vi "PolhemusTesting.vi"() -> ()   [LabVIEW 2009]
panel:
  out "roll":sgl format="%8.1f"
  out "el":sgl format="%8.1f"
  out "az":sgl format="%8.1f"
  in  "stop":bool
  out "z":sgl format="%8.1f"
  out "y":sgl format="%8.1f"
  out "x":sgl format="%8.1f"
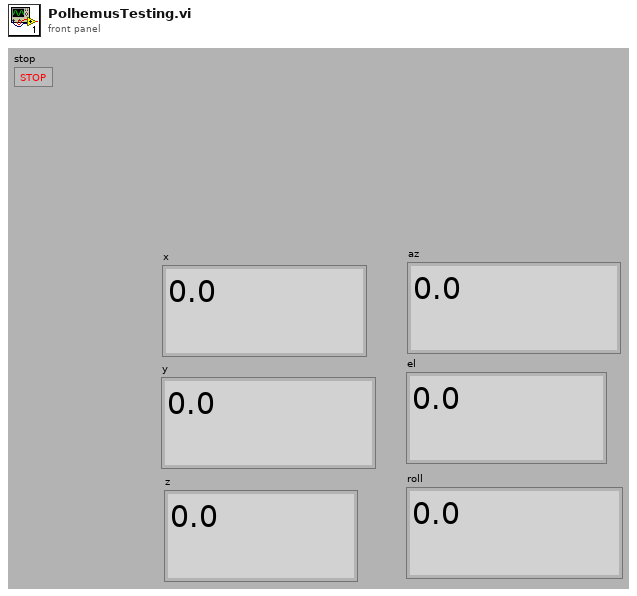
[diagram p1: front panel]
types:
  T1 = cluster{"#Bytes":i32[], "Titles":string[], "Format":enum16{"ASCII", "Binary"}, "Units":enum16{"Inches", "Centimeters"}, "Station State":bool[], "#Line Feeds":i32}
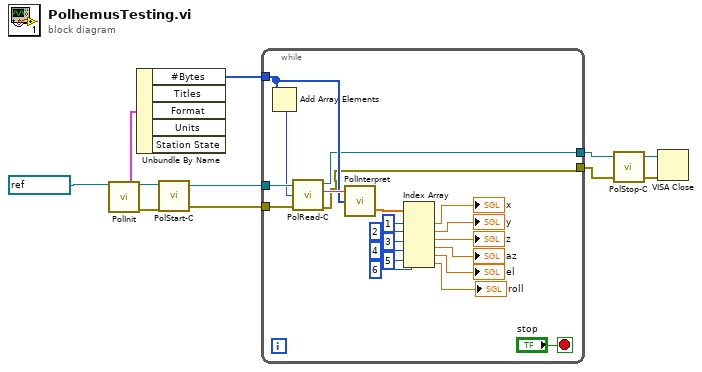
[diagram p0: block diagram]
diagram:
  n1 = call "PolInit.vi"("VISA resource name"=refnum<visa-resource-name> "COM3") -> ("VISA resource name out"=w9:refnum<visa-resource-name>, "Polhemus Info"=w10:T1, "error out"=w8:errorcluster)  [unwired: 12 in]
  n2 = Unbundle By Name(w10) -> ("#Bytes"=w5:i32[])  [unwired: 4 out]
  n3 = call "PolStart-C.vi"("error in (no error)"=w8, "VISA resource name"=w9) -> ("error out"=w6:errorcluster, "VISA resource name out"=w7:refnum<visa-resource-name>)  [unwired: 2 in]
  n4 = while {
    tunnel: w7 -> [w32]
    tunnel: w6 -> [w31]
    tunnel: w5 -> [w28]
    tunnel: [w20] -> w4
    tunnel: [w19] -> w3
    stop <- "stop" stop-if-true
    n5 = Add Array Elements(numeric array=w28) -> (sum=w30:i32)
    n6 = call "PolRead-C.vi"("VISA resource name"=w32, "Byte Sum"=w30, "error in (no error)"=w31) -> ("VISA resource name out"=w20:refnum<visa-resource-name>, "Polhemus Output"=w29:string, "error out"=w19:errorcluster)  [unwired: 1 out]
    n7 = call "PolInterpret.vi"("#Bytes"=w28, "Polhemus Output"=w29) -> ("Interpreted Values"=w27:sgl[])  [unwired: 2 in, 1 out]
    n8 = Index Array(array=w27, index #1=1 ("index"), index #2=2 ("index"), index #3=3 ("index"), index #4=4 ("index"), index #5=5 ("index"), index #6=6 ("index")) -> (element #1=→"x":sgl, element #2=→"y":sgl, element #3=→"z":sgl, element #4=→"az":sgl, element #5=→"el":sgl, element #6=→"roll":sgl)
  }
  n9 = call "PolStop-C.vi"("error in (no error)"=w3, "VISA resource name"=w4) -> ("error out"=w1:errorcluster, "VISA resource name out"=w2:refnum<visa-resource-name>)  [unwired: 2 in]
  n10 = VISA Close(VISA resource name=w2, error in (no error)=w1) -> ()  [unwired: 1 out]
